vi "Create Linked List.vi"(8 "error in (no error)":errorcluster, 11 "Linked List":refnum<class "ILinked List.lvclass">) -> (0 "error out":errorcluster, 3 "Linked List Ref":refnum<data-value>)   [LabVIEW 2017, in "Linked Lists.lvlib" / "Linked List Ref.lvclass"]
uses:
  <vilib>/gpm_packages/@cs/linked-list/Source/Linked List/Linked List Ref/Linked List Ref.lvclass
  <vilib>/gpm_packages/@cs/linked-list/Source/Linked List/ILinkedList/ILinked List.lvclass
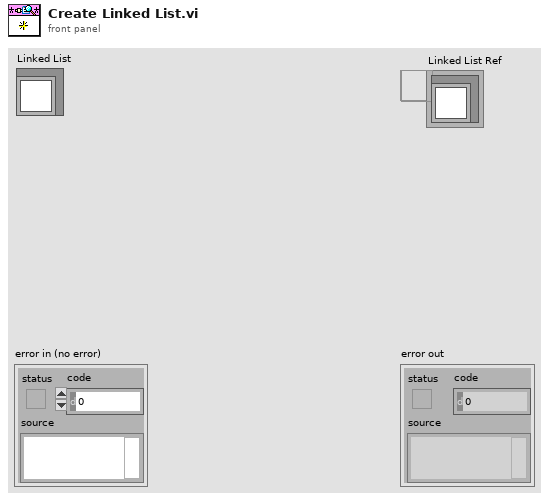
[diagram p1: front panel]
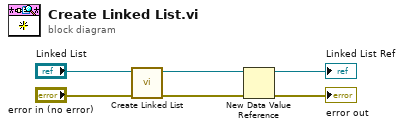
[diagram p0: block diagram]
diagram:
  n1 = call-dynamic "Create Linked List.vi"("error in (no error)"="error in (no error)", "ILinked List in"="Linked List") -> ("error out"=w2:errorcluster, "ILinked List out"=w1:refnum<class "ILinked List.lvclass">)  [unwired: 8 in]
  n2 = New Data Value Reference(data value=w1, error in=w2) -> (data value reference=→"Linked List Ref":refnum<data-value>, error out=→"error out":errorcluster)
